vi "Timed Loop Demo.vi"() -> ()   [LabVIEW 2015]
uses:
  <vilib>/Platform/TimedLoop/XDataNode/timing_clust.ctl
  <vilib>/Platform/TimedLoop/XDataNode/nitl_modes.ctl
  <vilib>/Platform/TimedLoop/XDataNode/wakeup.ctl
  <vilib>/Platform/TimedLoop/XDataNode/XDataNode.xnode
  <vilib>/Platform/TimedLoop/XDataNode/XDNodeRunTimeDep.lvlib
panel:
  out "Finished Late? [i-1]":bool
  out "Numeric":i32
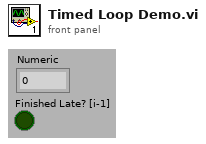
[diagram p1: front panel]
types:
  T1 = typedef "XDNodeRunTimeDep.lvlib/timing_clust.ctl" = cluster{"Expected End [f-1]":u64, "Actual End [f-1]":u64, "Finished Late? [f-1]":bool, "Expected End [i-1]":u64, "Actual End [i-1]":u64, "Finished Late? [i-1]":bool, "Expected Start [i]":u64, "Actual Start [i]":u64, "Expected Start [f]":u64, "Actual Start [f]":u64, "Source Name":string, "Structure Name":string, "Period":i64, "Deadline":i64, "Offset":i64, "Start":i64, "Priority":i32, "Timeout":i32, "Mode":T2, "Wakeup Reason":T3, "Error":errorcluster, "Source Type":string, "Secondary Source Type":string, "Global End Time":u64, "Global Start Time":u64, "Frame Duration":u64, "Iteration Duration":u64, "Assigned CPU":i32, "I/O Scan Engine Mode":u32}
  T2 = typedef "XDNodeRunTimeDep.lvlib/nitl_modes.ctl" = enum32{"No Change", "Process missed periods, maintain original phase", "Discard missed periods, maintain original phase", "Process missed periods, ignore original phase", "Discard missed periods, ignore original phase"}
  T3 = typedef "XDNodeRunTimeDep.lvlib/wakeup.ctl" = enum32{"Normal", "Aborted", "Asynchronous wakeup", "Timing source error", "Timed loop error", "Timeout"}
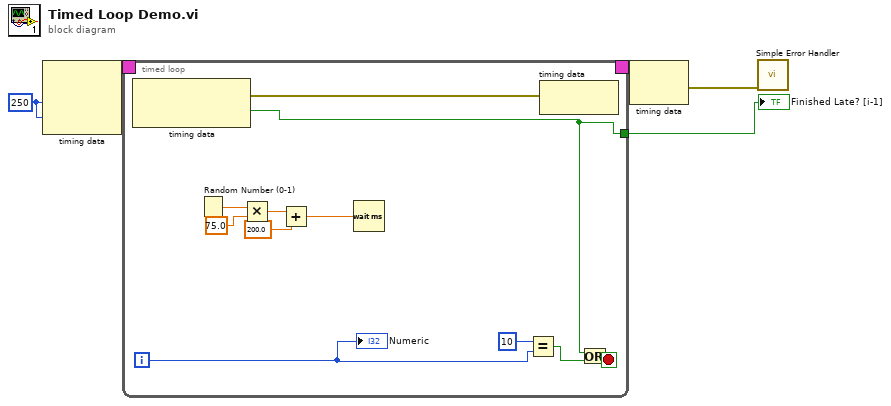
[diagram p0: block diagram]
diagram:
  w2 = i64 250 ("Period")
  n1 = node-c288(w2, w2) -> (w5:T1)  [unwired: 1 in]
  n2 = timed-loop {
    timing: w5 -> [_]
    timing-out: [_] -> w4
    tunnel: [w6] -> w1
    i -> [w16]
    stop <- w8 stop-if-true
    n3 = node-c288() -> (w14:errorcluster, w6:bool)  [unwired: 1 in]
    n4 = Random Number (0-1)() -> (number: 0 to 1=w13:dbl)
    n5 = Multiply(x=w13, y=75.0) -> (x*y=w12:dbl)
    n6 = Add(x=w12, y=200.0) -> (x+y=w11:dbl)
    n7 = Wait (ms)(milliseconds to wait=w11) -> ()  [unwired: 1 out]
    n8 = Equal?(x=10, y=w16) -> (x = y?=w7:bool)
    n9 = node-c288(w14) -> ()  [unwired: 1 out]
    n10 = Or(x=w6, y=w7) -> (x .or. y?=w8:bool)
    "Numeric" <- w16
  }
  "Finished Late? [i-1]" <- w1
  n11 = node-c288(w4) -> (w3:errorcluster)
  n12 = call <vilib>:"Simple Error Handler.vi"("error in (no error)"=w3) -> ()  [unwired: 4 in, 5 out]
